vi "Encoder Driver-messages module.vi"(8 "error in (no error)":errorcluster, 11 "Command/Response string":string) -> (0 "error":errorcluster)   [LabVIEW 2013]
uses:
  Globals/Encoder globals.vi
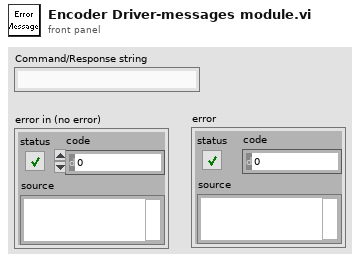
[diagram p1: front panel]
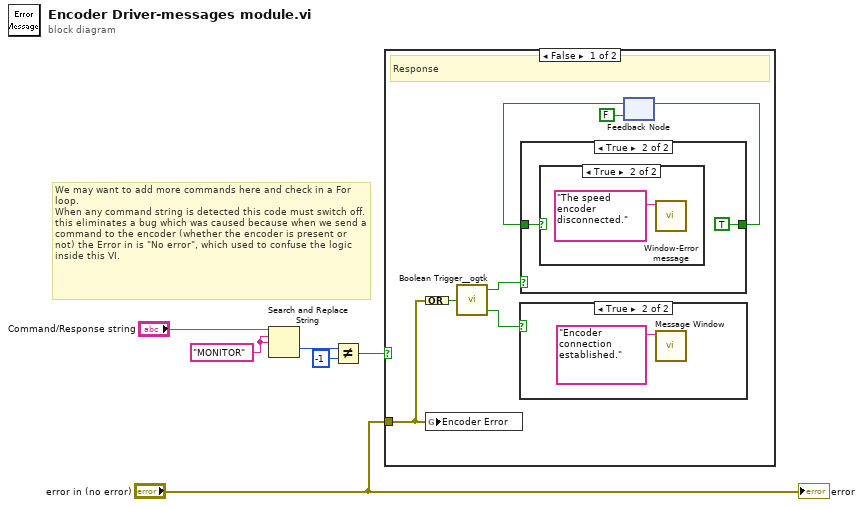
[diagram p0: block diagram]
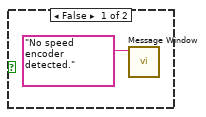
[diagram p3: hidden frame]
diagram:
  w5 = "MONITOR" ("data in")
  # "We may want to add more commands here and check in a For loop.\nWhen any command string is detected this code must switch off. this eliminates a bug which was caused because when we send a command to the encoder (whether the encoder is present or not) the Error in is \"No error\", which used to confuse the logic inside this VI."
  n1 = Search and Replace String(input string="Command/Response string", search string=w5, replace string=w5) -> (offset past replacement=w4:i32)  [unwired: 5 in, 3 out]
  n2 = Not Equal?(x=w4, y=-1) -> (x != y?=w2:bool)
  n3 = case shown="False" w2 {
    tunnel: "error in (no error)" -> [w7 _]
    frame False {
      # "Response"
      n4 = Compound Arithmetic op=OR(w7) -> (w12:bool)
      n5 = global write "Encoder globals.vi" "Encoder Error"(w7) -> ()
      n6 = call "Boolean Trigger__ogtk.vi"("Boolean Input"=w12) -> ("Rising Edge"=w13:bool, "Falling Edge"=w11:bool)  [unwired: 1 in]
      n7 = case shown="True" w11 {
        frame False {
        }
        frame True {
          n8 = call "Message Window.vi"("Message string"="Encoder connection established." ("Error Source")) -> ()  [unwired: 10 in, 1 out]
        }
      }
      n9 = feedback #1(FALSE) -> (w9:bool)
      n10 = case shown="True" w13 {
        tunnel: [w14 TRUE] -> w10
        tunnel: w9 -> [w14 w15]
        frame False {
        }
        frame True {
          n11 = case shown="True" w15 {
            frame False {
              n12 = call "Message Window.vi"("Message string"="No speed encoder detected." ("Error Source")) -> ()  [unwired: 10 in, 1 out]
            }
            frame True {
              n13 = call "Window-Error message.vi"("Message"="The speed encoder disconnected." ("Error Source")) -> ()  [unwired: 10 in, 1 out]
            }
          }
        }
      }
      n14 = feedback-in #1(w10) -> ()
    }
    frame True {
      # "Command"
    }
  }
  "error" <- "error in (no error)"
